vi "EX5 with EVENT STRUCTURE.vi"() -> ()   [LabVIEW 2018]
panel:
  out "date string":string
  out "time string":string
  in  "A":dbl
  in  "B":dbl
  out "Result":dbl
  in  "Operation":T1(ring)
  in  "stop":bool
  in  "Blank Button":bool
  # "EX5 avec ES - TP0"
  # "Mekni Marwen 2ème Année Génie Electrique"
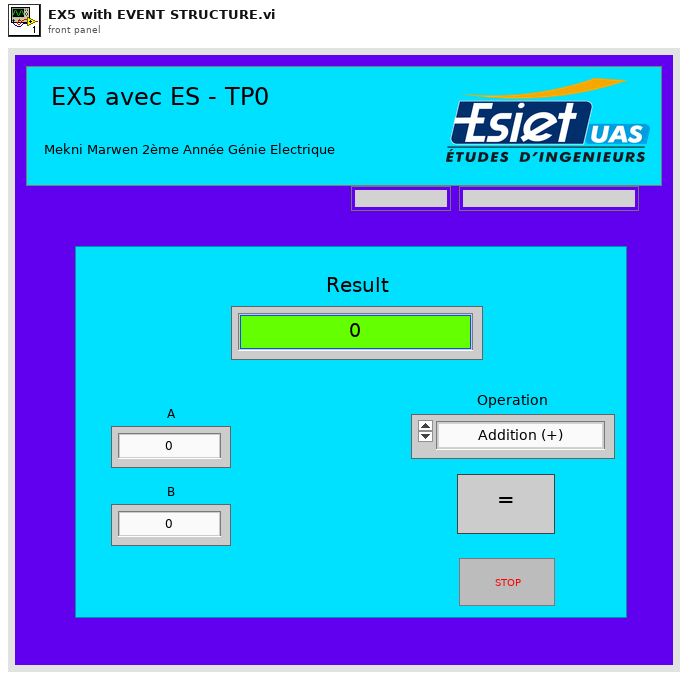
[diagram p1: front panel]
types:
  T1 = enum16{"Addition (+)", "Subtraction (-)", "Multiplication (×)", "Division (÷)"}
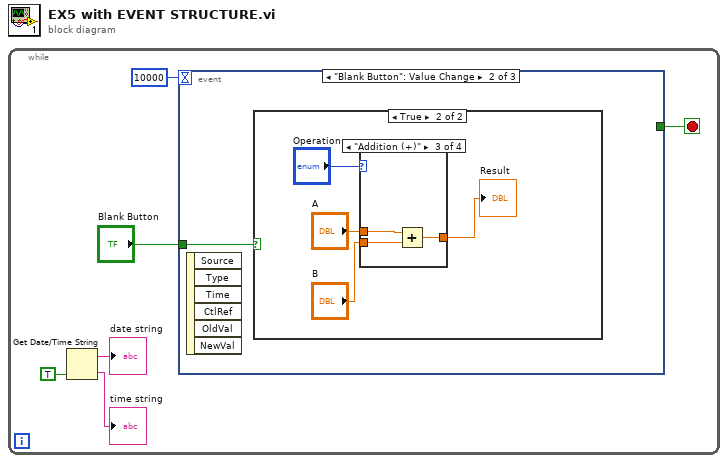
[diagram p0: block diagram]
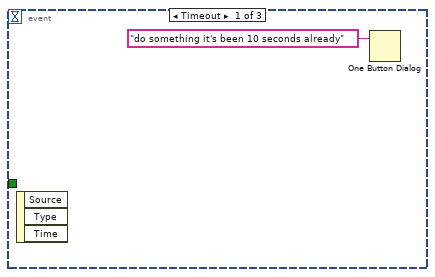
[diagram p2: hidden frame]
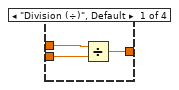
[diagram p4: hidden frame]
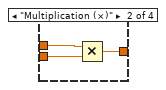
[diagram p5: hidden frame]
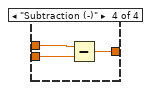
[diagram p6: hidden frame]
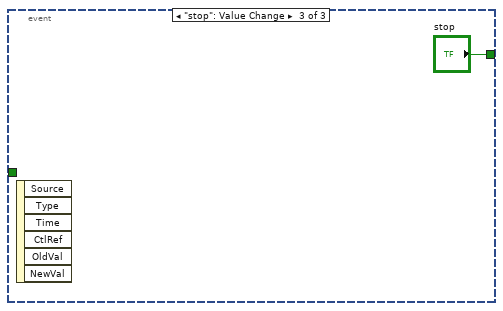
[diagram p7: hidden frame]
diagram:
  n1 = while {
    stop <- w5 stop-if-true
    n2 = Get Date/Time String(want seconds? (F)=TRUE) -> (date string=→"date string":string, time string=→"time string":string)  [unwired: 2 in]
    n3 = event shown="[1] \"Blank Button\": Value Change" {
      selector: _ -> [_ _ _]
      dyn-events: _ -> [_ _ _]
      timeout: 10000 -> [_ _ _]
      tunnel: [_ _ "stop"] -> w5
      tunnel: "Blank Button" -> [_ w8 _]
      event Timeout {
        n4 = event-data() -> ()  [unwired: 1 in, 3 out]
        n5 = One Button Dialog(message="do something it's been 10 seconds already") -> ()  [unwired: 1 in, 1 out]
      }
      event "Blank Button": Value Change {
        n6 = event-data() -> ()  [unwired: 1 in, 6 out]
        n7 = case shown="True" w8 {
          frame False {
          }
          frame True {
            n8 = case shown="\"Addition (+)\"" "Operation" {
              tunnel: "A" -> [w15 w18 w20 w23]
              tunnel: "B" -> [w14 w17 w19 w22]
              tunnel: [w13 w16 w21 w24] -> w9
              frame "Division (÷)", Default {
                n9 = Divide(x=w15, y=w14) -> (x/y=w13:dbl)
              }
              frame "Multiplication (×)" {
                n10 = Multiply(x=w18, y=w17) -> (x*y=w16:dbl)
              }
              frame "Addition (+)" {
                n11 = Add(x=w20, y=w19) -> (x+y=w21:dbl)
              }
              frame "Subtraction (-)" {
                n12 = Subtract(x=w23, y=w22) -> (x-y=w24:dbl)
              }
            }
            "Result" <- w9
          }
        }
      }
      event "stop": Value Change {
        n13 = event-data() -> ()  [unwired: 1 in, 6 out]
      }
    }
  }
